vi "LogicSNRvariations.vi"() -> ()   [LabVIEW 2012]
panel:
  in  "Frequency of\noperation":dbl
  out "Required SNR":dbl
  in  "Modulation":dbl
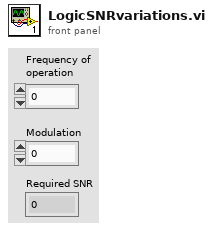
[diagram p1: front panel]
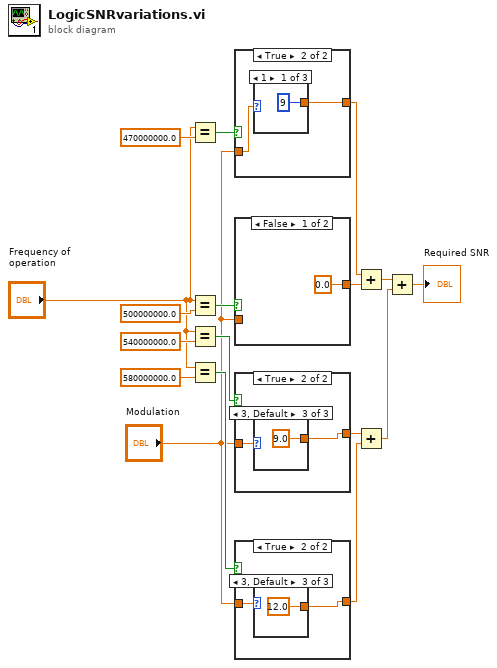
[diagram p0: block diagram]
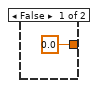
[diagram p2: hidden frame]
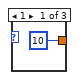
[diagram p3: hidden frame]
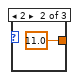
[diagram p4: hidden frame]
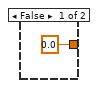
[diagram p5: hidden frame]
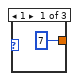
[diagram p6: hidden frame]
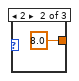
[diagram p7: hidden frame]
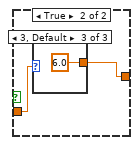
[diagram p8: hidden frame]
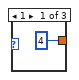
[diagram p9: hidden frame]
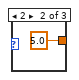
[diagram p10: hidden frame]
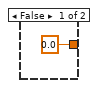
[diagram p11: hidden frame]
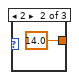
[diagram p12: hidden frame]
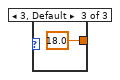
[diagram p13: hidden frame]
diagram:
  n1 = Equal?(x="Frequency of\noperation", y=470000000.0) -> (x = y?=w3:bool)
  n2 = Equal?(x="Frequency of\noperation", y=500000000.0) -> (x = y?=w4:bool)
  n3 = Equal?(x="Frequency of\noperation", y=540000000.0) -> (x = y?=w5:bool)
  n4 = Equal?(x="Frequency of\noperation", y=580000000.0) -> (x = y?=w6:bool)
  n5 = case shown="True" w3 {
    tunnel: [0.0 w19] -> w14
    tunnel: "Modulation" -> [_ w20]
    frame False {
    }
    frame True {
      n6 = case shown="1" w20 {
        tunnel: [9 14.0 18.0] -> w19
        frame 1 {
        }
        frame 2 {
        }
        frame 3, Default {
        }
      }
    }
  }
  n7 = case shown="False" w4 {
    tunnel: [0.0 w25] -> w13
    tunnel: "Modulation" -> [_ w26]
    frame False {
    }
    frame True {
      n8 = case shown="3, Default" w26 {
        tunnel: [4 5.0 6.0] -> w25
        frame 1 {
        }
        frame 2 {
        }
        frame 3, Default {
        }
      }
    }
  }
  n9 = case shown="True" w5 {
    tunnel: [0.0 w31] -> w12
    tunnel: "Modulation" -> [_ w32]
    frame False {
    }
    frame True {
      n10 = case shown="3, Default" w32 {
        tunnel: [7 8.0 9.0] -> w31
        frame 1 {
        }
        frame 2 {
        }
        frame 3, Default {
        }
      }
    }
  }
  n11 = case shown="True" w6 {
    tunnel: [0.0 w37] -> w11
    tunnel: "Modulation" -> [_ w38]
    frame False {
    }
    frame True {
      n12 = case shown="3, Default" w38 {
        tunnel: [10 11.0 12.0] -> w37
        frame 1 {
        }
        frame 2 {
        }
        frame 3, Default {
        }
      }
    }
  }
  n13 = Add(x=w14, y=w13) -> (x+y=w17:dbl)
  n14 = Add(x=w12, y=w11) -> (x+y=w16:dbl)
  n15 = Add(x=w17, y=w16) -> (x+y=→"Required SNR":dbl)
